vi "Monta Comando FOCO.vi"(5 "IN":bool=TRUE, 6 "Set Point":string, 7 "Comando":string, 8 "Dispositivo":string, 9 "Controlador":u16(ring)=1 items=["ZERO", "AH", "DEC", "TUBO", "CUP"]) -> (0 "Erro Comunicação":bool, 1 "String Enviado":string, 2 "Resposta":string)   [LabVIEW 2018]
uses:
  Global_Telescopio.vi
panel:
  out "Numeric":i32
  out "Erro Resp":bool
  out "ERRO":bool
  out "String Enviado":string
  # "PROG"
  # "SIDERAL"
  # "EMBREAGEM"
  # "DESLIGAR"
  # "STATUS"
  # "LIGAR"
  # "PARAR"
  # "ERROS"
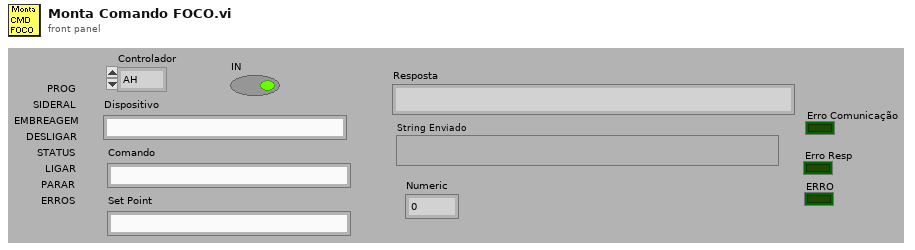
[diagram p1: front panel]
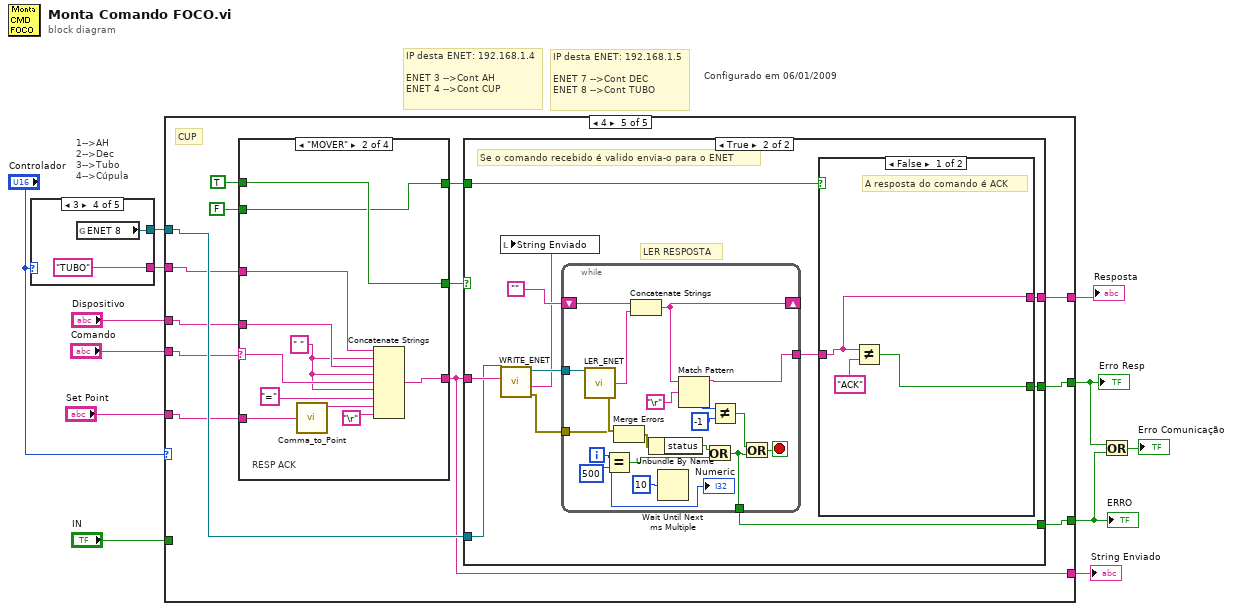
[diagram p0: block diagram]
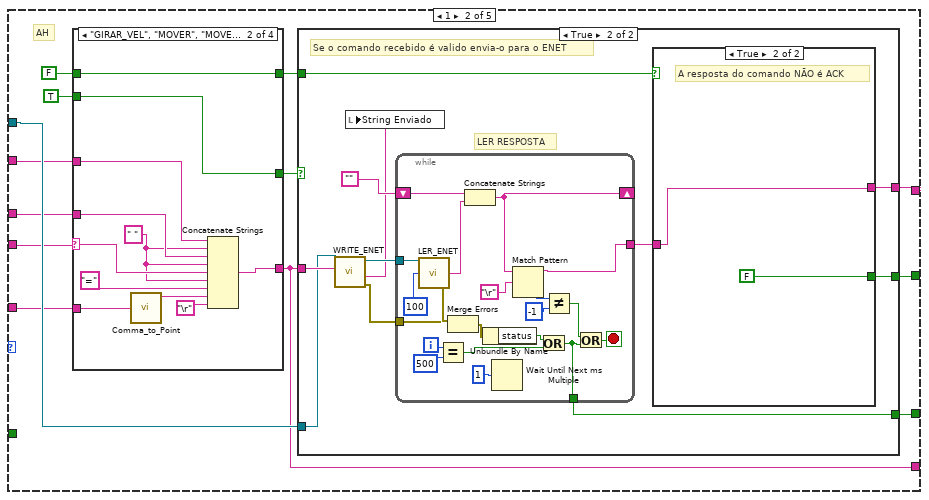
[diagram p3: hidden frame]
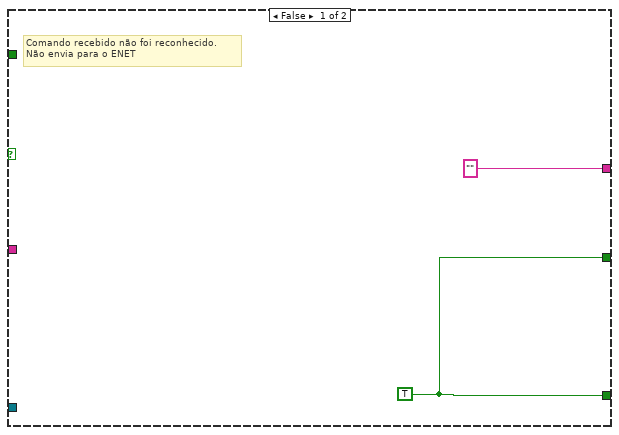
[diagram p4: hidden frame]
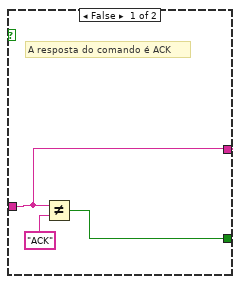
[diagram p5: hidden frame]
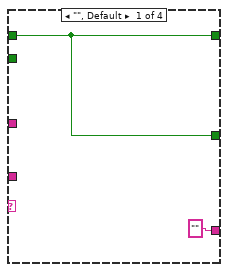
[diagram p6: hidden frame]
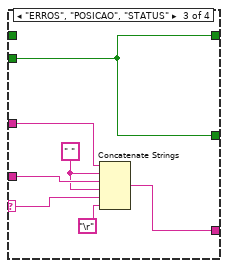
[diagram p7: hidden frame]
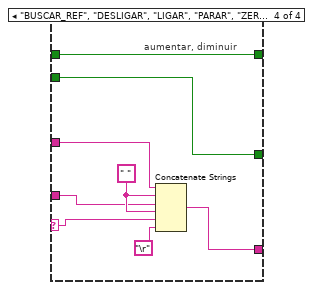
[diagram p8: hidden frame]
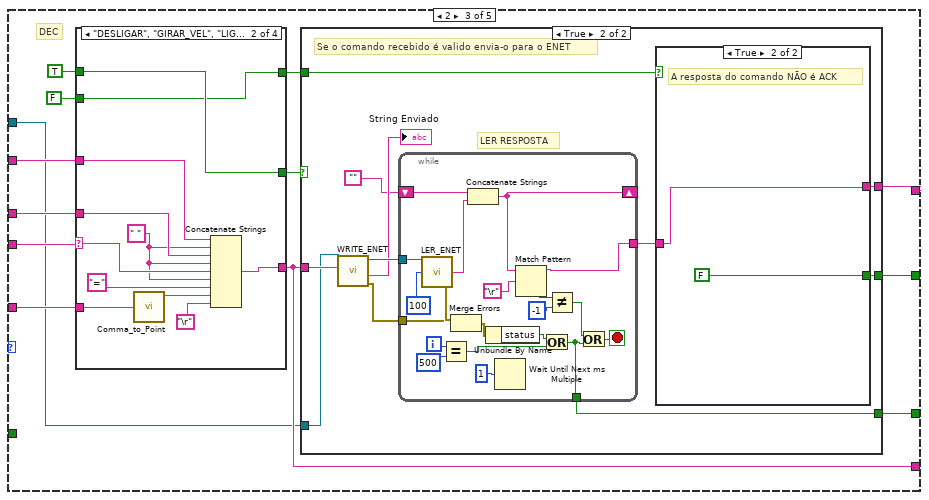
[diagram p9: hidden frame]
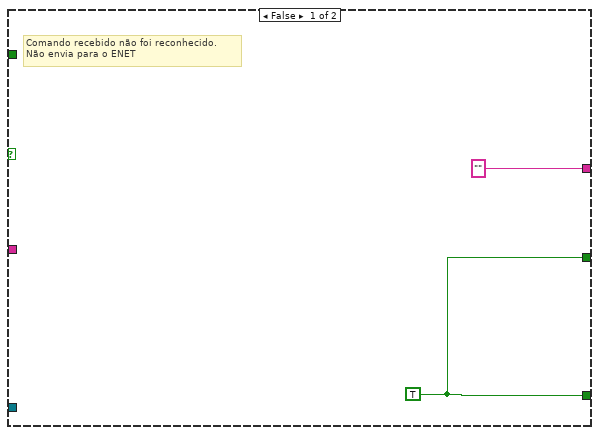
[diagram p10: hidden frame]
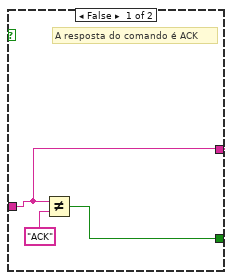
[diagram p11: hidden frame]
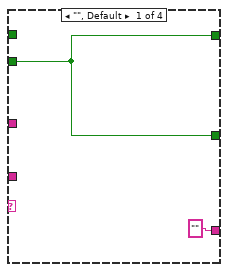
[diagram p12: hidden frame]
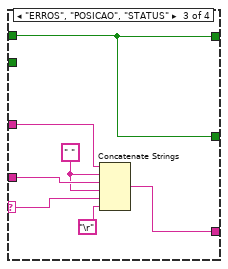
[diagram p13: hidden frame]
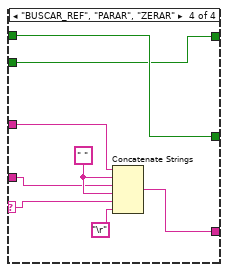
[diagram p14: hidden frame]
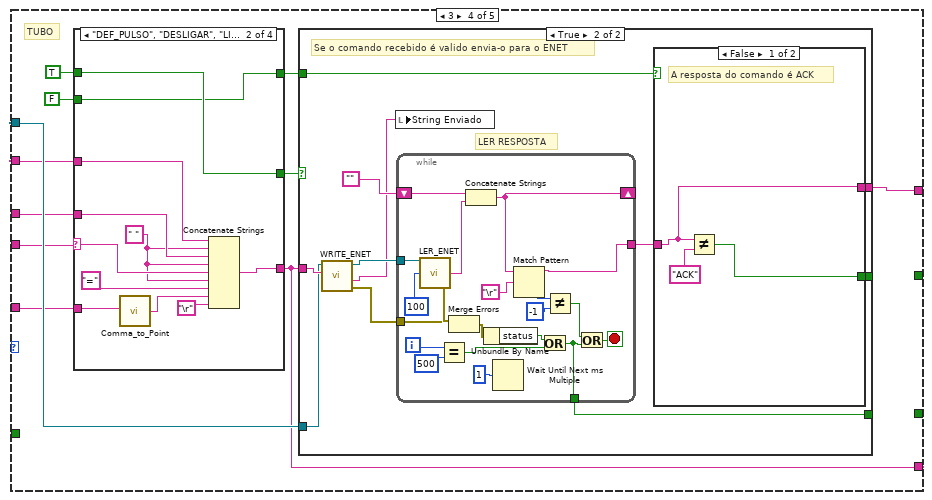
[diagram p15: hidden frame]
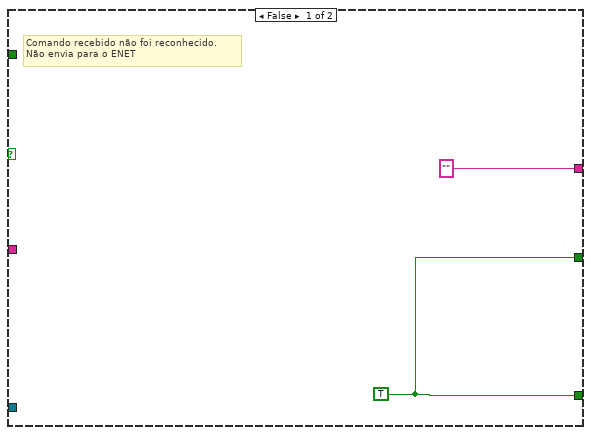
[diagram p16: hidden frame]
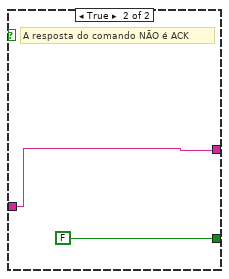
[diagram p17: hidden frame]
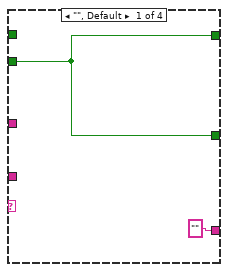
[diagram p18: hidden frame]
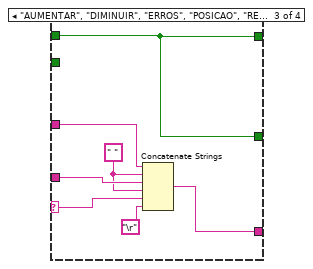
[diagram p19: hidden frame]
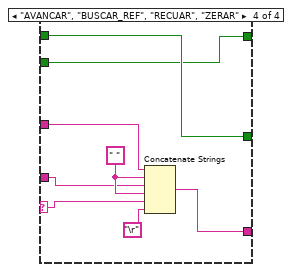
[diagram p20: hidden frame]
diagram:
  # "Configurado em 06/01/2009"
  # "IP desta ENET: 192.168.1.4\n\nENET 3 -->Cont AH\nENET 4 -->Cont CUP"
  # "IP desta ENET: 192.168.1.5\n\nENET 7 -->Cont DEC\nENET 8 -->Cont TUBO"
  # "1-->AH\n2-->Dec\n3-->Tubo\n4-->Cúpula"
  n1 = case shown="3" "Controlador" {
    tunnel: ["ZERO" ("string") "AH" ("string") "DEC" ("string") "TUBO" ("string") "CUP" ("string")] -> w8
    tunnel: [w13 w15 w17 w19 w21] -> w6
    frame 0, Default {
      n2 = global read "Global_Telescopio.vi" "ENET 3"() -> (w13:refnum<visa-resource-name>)
    }
    frame 1 {
      n3 = global read "Global_Telescopio.vi" "ENET 3"() -> (w15:refnum<visa-resource-name>)
    }
    frame 2 {
      n4 = global read "Global_Telescopio.vi" "ENET 7"() -> (w17:refnum<visa-resource-name>)
    }
    frame 3 {
      n5 = global read "Global_Telescopio.vi" "ENET 8"() -> (w19:refnum<visa-resource-name>)
    }
    frame 4 {
      n6 = global read "Global_Telescopio.vi" "ENET 4"() -> (w21:refnum<visa-resource-name>)
    }
  }
  n7 = case shown="4" "Controlador" {
    tunnel: "Dispositivo" -> [_ w29 w114 w185 w264]
    tunnel: "Comando" -> [_ w28 w112 w184 w263]
    tunnel: "Set Point" -> [_ w27 w113 w183 w262]
    tunnel: w8 -> [_ w30 w111 w186 w265]
    tunnel: [_ w23 w106 w181 w259] -> w7
    tunnel: [_ w25 w104 _ w258] -> w4
    tunnel: [_ w24 w103 _ w260] -> w5
    tunnel: w6 -> [_ w31 w102 w187 w266]
    tunnel: "IN" -> [_ _ _ _ _]
    tunnel: [_ w26 w105 w182 w261] -> w1
    frame 0, Default {
      # "ZERO"
    }
    frame 1 {
      # "AH"
      n8 = case shown="\"GIRAR_VEL\", \"MOVER\", \"MOVER_ABS\", \"MOVER_RAP\", \"MOVER_REL\", \"VAR_TRACK\"" w28 {
        selector: w28 -> [_ w83 w90 w96]
        tunnel: w29 -> [_ w86 w91 w97]
        tunnel: w27 -> [_ w85 _ _]
        tunnel: ["" w84 w92 w99] -> w26
        tunnel: w30 -> [_ w82 w88 w98]
        tunnel: [w74 w81 w87 w95] -> w35
        tunnel: FALSE -> [w74 w80 _ w94]
        tunnel: TRUE -> [_ w81 w87 w95]
        tunnel: [w74 w80 w87 w94] -> w32
        frame "", Default {
        }
        frame "GIRAR_VEL", "MOVER", "MOVER_ABS", "MOVER_RAP", "MOVER_REL", "VAR_TRACK" {
          w79 = " "
          n9 = call "Comma_to_Point.vi"("Lat_A"=w85) -> ("Saída"=w77:string)
          n10 = Concatenate Strings(w82, w79, w86, w79, w83, w79, "=", w77, "\r") -> (w84:string)
        }
        frame "ERROS", "POSICAO", "STATUS" {
          w89 = " "
          n11 = Concatenate Strings(w88, w89, w91, w89, w90, "\r") -> (w92:string)
        }
        frame "BUSCAR_REF", "DESLIGAR", "LIGAR", "PARAR", "ZERAR" {
          w100 = " "
          # "aumentar, diminuir"
          n12 = Concatenate Strings(w98, w100, w97, w100, w96, "\r") -> (w99:string)
        }
      }
      n13 = case shown="True" w35 {
        tunnel: ["" w43] -> w23
        tunnel: w26 -> [_ w46]
        tunnel: w32 -> [_ w44]
        tunnel: [w36 w42] -> w25
        tunnel: [w36 w41] -> w24
        tunnel: w31 -> [_ w40]
        frame False {
          w36 = TRUE
          # "Comando recebido não foi reconhecido.\nNão envia para o ENET"
        }
        frame True {
          # "LER RESPOSTA"
          # "Se o comando recebido é valido envia-o para o ENET"
          n14 = call "WRITE_ENET.vi"("String a ser Enviado"=w46, "LNA VISA session (for class)"=w40) -> ("error out"=w47:errorcluster, "String Enviado"=w39:string, "LNA VISA session saida"=w48:refnum<visa-resource-name>)  [unwired: 3 in]
          n15 = local write "String Enviado"(w39) -> ()
          n16 = while {
            tunnel: w48 -> [w73]
            tunnel: w47 -> [w70]
            tunnel: [w54] -> w38
            shift-right: [w56] -> _
            shift-left: "" -> [w58]
            tunnel: [w55] -> w42
            i -> [w64]
            stop <- w59 stop-if-true
            n17 = call "LER_ENET.vi"("Num de Bytes a Ser lido"=u32 100, "LNA VISA resource name"=w73) -> ("error out"=w71:errorcluster, "String Lida"=w57:string)  [unwired: 1 in, 1 out]
            n18 = Equal?(x=w64, y=500) -> (x = y?=w62:bool)
            n19 = Merge Errors(w71, w70) -> (w69:errorcluster)
            n20 = Concatenate Strings(w58, w57) -> (w56:string)
            n21 = Unbundle By Name(w69) -> ("status"=w61:bool)
            n22 = Wait Until Next ms Multiple(millisecond multiple=u32 1) -> ()  [unwired: 1 out]
            n23 = Match Pattern(string=w56, regular expression="\r") -> (before substring=w54:string, offset past match=w66:i32)  [unwired: 1 in, 2 out]
            n24 = Or(x=w61, y=w62) -> (x .or. y?=w55:bool)
            n25 = Not Equal?(x=w66, y=-1) -> (x != y?=w60:bool)
            n26 = Or(x=w60, y=w55) -> (x .or. y?=w59:bool)
          }
          n27 = case shown="True" w44 {
            tunnel: w38 -> [w50 w52]
            tunnel: [w50 w52] -> w43
            tunnel: [w49 FALSE] -> w41
            frame False {
              # "A resposta do comando é ACK"
              n28 = Not Equal?(x=w50, y="ACK") -> (x != y?=w49:bool)
            }
            frame True {
              # "A resposta do comando NÃO é ACK"
            }
          }
        }
      }
    }
    frame 2 {
      # "DEC"
      n29 = case shown="\"DESLIGAR\", \"GIRAR_VEL\", \"LIGAR\", \"MOVER_ABS\", \"MOVER_RAP\", \"MOVER_REL\", \"VAR_TRACK\"" w112 {
        selector: w112 -> [_ w162 w169 w175]
        tunnel: w114 -> [_ w165 w170 w176]
        tunnel: w113 -> [_ w164 _ _]
        tunnel: ["" w163 w171 w178] -> w105
        tunnel: w111 -> [_ w161 w167 w177]
        tunnel: [w153 w160 w166 w174] -> w110
        tunnel: FALSE -> [w153 w159 _ w173]
        tunnel: TRUE -> [_ w160 w166 w174]
        tunnel: [w153 w159 w166 w173] -> w107
        frame "", Default {
        }
        frame "DESLIGAR", "GIRAR_VEL", "LIGAR", "MOVER_ABS", "MOVER_RAP", "MOVER_REL", "VAR_TRACK" {
          w158 = " "
          n30 = call "Comma_to_Point.vi"("Lat_A"=w164) -> ("Saída"=w156:string)
          n31 = Concatenate Strings(w161, w158, w165, w158, w162, w158, "=", w156, "\r") -> (w163:string)
        }
        frame "ERROS", "POSICAO", "STATUS" {
          w168 = " "
          n32 = Concatenate Strings(w167, w168, w170, w168, w169, "\r") -> (w171:string)
        }
        frame "BUSCAR_REF", "PARAR", "ZERAR" {
          w179 = " "
          n33 = Concatenate Strings(w177, w179, w176, w179, w175, "\r") -> (w178:string)
        }
      }
      n34 = case shown="True" w110 {
        tunnel: ["" w121] -> w106
        tunnel: w105 -> [_ w124]
        tunnel: w107 -> [_ w122]
        tunnel: [w115 w120] -> w104
        tunnel: [w115 w119] -> w103
        tunnel: w102 -> [_ w118]
        frame False {
          w115 = TRUE
          # "Comando recebido não foi reconhecido.\nNão envia para o ENET"
        }
        frame True {
          # "LER RESPOSTA"
          # "Se o comando recebido é valido envia-o para o ENET"
          n35 = call "WRITE_ENET.vi"("String a ser Enviado"=w124, "LNA VISA session (for class)"=w118) -> ("error out"=w125:errorcluster, "String Enviado"=→"String Enviado":string, "LNA VISA session saida"=w127:refnum<visa-resource-name>)  [unwired: 3 in]
          n36 = while {
            tunnel: w127 -> [w152]
            tunnel: w125 -> [w149]
            tunnel: [w136] -> w117
            shift-right: [w134] -> _
            shift-left: "" -> [w137]
            tunnel: [w133] -> w120
            i -> [w143]
            stop <- w138 stop-if-true
            n37 = call "LER_ENET.vi"("Num de Bytes a Ser lido"=u32 100, "LNA VISA resource name"=w152) -> ("error out"=w150:errorcluster, "String Lida"=w135:string)  [unwired: 1 in, 1 out]
            n38 = Equal?(x=w143, y=500) -> (x = y?=w141:bool)
            n39 = Merge Errors(w150, w149) -> (w148:errorcluster)
            n40 = Concatenate Strings(w137, w135) -> (w134:string)
            n41 = Unbundle By Name(w148) -> ("status"=w140:bool)
            n42 = Wait Until Next ms Multiple(millisecond multiple=u32 1) -> ()  [unwired: 1 out]
            n43 = Match Pattern(string=w134, regular expression="\r") -> (before substring=w136:string, offset past match=w145:i32)  [unwired: 1 in, 2 out]
            n44 = Or(x=w140, y=w141) -> (x .or. y?=w133:bool)
            n45 = Not Equal?(x=w145, y=-1) -> (x != y?=w139:bool)
            n46 = Or(x=w139, y=w133) -> (x .or. y?=w138:bool)
          }
          n47 = case shown="True" w122 {
            tunnel: w117 -> [w129 w131]
            tunnel: [w129 w131] -> w121
            tunnel: [w128 FALSE] -> w119
            frame False {
              # "A resposta do comando é ACK"
              n48 = Not Equal?(x=w129, y="ACK") -> (x != y?=w128:bool)
            }
            frame True {
              # "A resposta do comando NÃO é ACK"
            }
          }
        }
      }
    }
    frame 3 {
      # "TUBO"
      n49 = case shown="\"DEF_PULSO\", \"DESLIGAR\", \"LIGAR\", \"MOVER\", \"MOVER_ABS\", \"MOVER_RAP\", \"MOVER_REL\", \"PARAR\", \"VAR_TRACK\"" w184 {
        selector: w184 -> [_ w240 w246 w252]
        tunnel: w185 -> [_ w242 w247 w253]
        tunnel: w183 -> [_ w232 _ _]
        tunnel: ["" w241 w248 w255] -> w182
        tunnel: w186 -> [_ w239 w244 w254]
        tunnel: [w230 w238 w243 w251] -> w191
        tunnel: FALSE -> [w230 w237 _ w250]
        tunnel: TRUE -> [_ w238 w243 w251]
        tunnel: [w230 w237 w243 w250] -> w188
        frame "", Default {
        }
        frame "DEF_PULSO", "DESLIGAR", "LIGAR", "MOVER", "MOVER_ABS", "MOVER_RAP", "MOVER_REL", "PARAR", "VAR_TRACK" {
          w236 = " "
          n50 = call "Comma_to_Point.vi"("Lat_A"=w232) -> ("Saída"=w233:string)
          n51 = Concatenate Strings(w239, w236, w242, w236, w240, w236, "=", w233, "\r") -> (w241:string)
        }
        frame "AUMENTAR", "DIMINUIR", "ERROS", "POSICAO", "REFINAR+", "REFINAR-", "STATUS" {
          w245 = " "
          n52 = Concatenate Strings(w244, w245, w247, w245, w246, "\r") -> (w248:string)
        }
        frame "AVANCAR", "BUSCAR_REF", "RECUAR", "ZERAR" {
          w256 = " "
          n53 = Concatenate Strings(w254, w256, w253, w256, w252, "\r") -> (w255:string)
        }
      }
      n54 = case shown="True" w191 {
        tunnel: ["" w202] -> w181
        tunnel: w182 -> [_ w198]
        tunnel: w188 -> [_ w203]
        tunnel: [w192 w201] -> _
        tunnel: [w192 w200] -> _
        tunnel: w187 -> [_ w197]
        frame False {
          w192 = TRUE
          # "Comando recebido não foi reconhecido.\nNão envia para o ENET"
        }
        frame True {
          # "LER RESPOSTA"
          # "Se o comando recebido é valido envia-o para o ENET"
          n55 = call "WRITE_ENET.vi"("String a ser Enviado"=w198, "LNA VISA session (for class)"=w197) -> ("error out"=w194:errorcluster, "String Enviado"=w195:string, "LNA VISA session saida"=w196:refnum<visa-resource-name>)  [unwired: 3 in]
          n56 = local write "String Enviado"(w195) -> ()
          n57 = while {
            tunnel: w196 -> [w229]
            tunnel: w194 -> [w226]
            tunnel: [w211] -> w199
            shift-right: [w213] -> _
            shift-left: "" -> [w215]
            tunnel: [w212] -> w201
            i -> [w220]
            stop <- w216 stop-if-true
            n58 = call "LER_ENET.vi"("Num de Bytes a Ser lido"=u32 100, "LNA VISA resource name"=w229) -> ("error out"=w227:errorcluster, "String Lida"=w214:string)  [unwired: 1 in, 1 out]
            n59 = Equal?(x=w220, y=500) -> (x = y?=w210:bool)
            n60 = Merge Errors(w227, w226) -> (w225:errorcluster)
            n61 = Concatenate Strings(w215, w214) -> (w213:string)
            n62 = Unbundle By Name(w225) -> ("status"=w218:bool)
            n63 = Wait Until Next ms Multiple(millisecond multiple=u32 1) -> ()  [unwired: 1 out]
            n64 = Match Pattern(string=w213, regular expression="\r") -> (before substring=w211:string, offset past match=w222:i32)  [unwired: 1 in, 2 out]
            n65 = Or(x=w218, y=w210) -> (x .or. y?=w212:bool)
            n66 = Not Equal?(x=w222, y=-1) -> (x != y?=w217:bool)
            n67 = Or(x=w217, y=w212) -> (x .or. y?=w216:bool)
          }
          n68 = case shown="False" w203 {
            tunnel: w199 -> [w206 w208]
            tunnel: [w206 w208] -> w202
            tunnel: [w205 FALSE] -> w200
            frame False {
              # "A resposta do comando é ACK"
              n69 = Not Equal?(x=w206, y="ACK") -> (x != y?=w205:bool)
            }
            frame True {
              # "A resposta do comando NÃO é ACK"
            }
          }
        }
      }
    }
    frame 4 {
      # "CUP"
      n70 = case shown="\"MOVER\"" w263 {
        selector: w263 -> [_ w317 w324 w330]
        tunnel: w264 -> [_ w320 w325 w331]
        tunnel: w262 -> [_ w319 _ _]
        tunnel: ["" w318 w326 w333] -> w261
        tunnel: w265 -> [_ w316 w322 w332]
        tunnel: [w308 w315 w321 w329] -> w270
        tunnel: FALSE -> [w308 w314 _ w328]
        tunnel: TRUE -> [_ w315 w321 w329]
        tunnel: [w308 w314 w321 w328] -> w267
        frame "", Default {
        }
        frame "MOVER" {
          w313 = " "
          # "RESP ACK"
          n71 = call "Comma_to_Point.vi"("Lat_A"=w319) -> ("Saída"=w311:string)
          n72 = Concatenate Strings(w316, w313, w320, w313, w317, w313, "=", w311, "\r") -> (w318:string)
        }
        frame "ERROS", "POSICAO", "STATUS" {
          w323 = " "
          # "RESP NÃO ACK"
          n73 = Concatenate Strings(w322, w323, w325, w323, w324, "\r") -> (w326:string)
        }
        frame "ABRIR", "DESCER", "FECHAR", "PARAR", "SUBIR" {
          w334 = " "
          # "ACK"
          n74 = Concatenate Strings(w332, w334, w331, w334, w330, "\r") -> (w333:string)
        }
      }
      n75 = case shown="True" w270 {
        tunnel: ["" w278] -> w259
        tunnel: w261 -> [_ w281]
        tunnel: w267 -> [_ w279]
        tunnel: [w271 w277] -> w258
        tunnel: [w271 w276] -> w260
        tunnel: w266 -> [_ w275]
        frame False {
          w271 = TRUE
          # "Comando recebido não foi reconhecido.\nNão envia para o ENET"
        }
        frame True {
          # "LER RESPOSTA"
          # "Se o comando recebido é valido envia-o para o ENET"
          n76 = call "WRITE_ENET.vi"("String a ser Enviado"=w281, "LNA VISA session (for class)"=w275) -> ("error out"=w282:errorcluster, "String Enviado"=w273:string, "LNA VISA session saida"=w283:refnum<visa-resource-name>)  [unwired: 3 in]
          n77 = local write "String Enviado"(w273) -> ()
          n78 = while {
            tunnel: w283 -> [w307]
            tunnel: w282 -> [w305]
            tunnel: [w293] -> w274
            shift-right: [w291] -> _
            shift-left: "" -> [w294]
            tunnel: [w290] -> w277
            i -> [w289]
            stop <- w295 stop-if-true
            n79 = call "LER_ENET.vi"("LNA VISA resource name"=w307) -> ("error out"=w306:errorcluster, "String Lida"=w292:string)  [unwired: 2 in, 1 out]
            n80 = Equal?(x=w289, y=500) -> (x = y?=w298:bool)
            n81 = Merge Errors(w306, w305) -> (w304:errorcluster)
            n82 = Concatenate Strings(w294, w292) -> (w291:string)
            n83 = Unbundle By Name(w304) -> ("status"=w297:bool)
            n84 = Wait Until Next ms Multiple(millisecond multiple=u32 10) -> ()  [unwired: 1 out]
            n85 = Match Pattern(string=w291, regular expression="\r") -> (before substring=w293:string, offset past match=w301:i32)  [unwired: 1 in, 2 out]
            n86 = Or(x=w297, y=w298) -> (x .or. y?=w290:bool)
            n87 = Not Equal?(x=w301, y=-1) -> (x != y?=w296:bool)
            n88 = Or(x=w296, y=w290) -> (x .or. y?=w295:bool)
            "Numeric" <- w289
          }
          n89 = case shown="False" w279 {
            tunnel: w274 -> [w285 w287]
            tunnel: [w285 w287] -> w278
            tunnel: [w284 FALSE] -> w276
            frame False {
              # "A resposta do comando é ACK"
              n90 = Not Equal?(x=w285, y="ACK") -> (x != y?=w284:bool)
            }
            frame True {
              # "A resposta do comando NÃO é ACK"
            }
          }
        }
      }
    }
  }
  "Resposta" <- w7
  "String Enviado" <- w1
  "ERRO" <- w4
  "Erro Resp" <- w5
  n91 = Or(x=w5, y=w4) -> (x .or. y?=→"Erro Comunicação":bool)
